vi "LTC change to stable temp.vi"(2 "Point Number":i32 min=-20 step=1, 3 "L:TC 21 Address":refnum<visa-resource-name>) -> (0 "Stop":bool, 1 "Stable temperature (K)":dbl[](array[numeric]) format="%.2f")   [LabVIEW 2025]
doc: "Changes the setpoint and waits for temperature to stablilize near the setpoint. Can set how stable and how close to the setpoint one wants the temperature to be. Allows changing of the PID parameters.\nMurali Chaparala, Scott Hannahs, NHMFL - FSU, November 1996\nAuthor: Scott Hannahs <sth@magnet.fsu.edu>\n\nThis software is licensed for use under the “MIT License\"\nCopyright (c) 2025 Scott Hannahs, sth@sth@magnet.sthnet.net\n\nPermission is hereby granted, free of charge, to any person obtaining a copy of this software and associated documentation files (the \"Software\"), to deal in the Software without restriction, including without limitation the rights to use, copy, modify, merge, publish, distribute, sublicense, and/or sell copies of the Software, and to permit persons to whom the Software is furnished to do so, subject to the following conditions: The above copyright notice and this permission notice shall be included in all copies or substantial portions of the Software.\n\nTHE SOFTWARE IS PROVIDED \"AS IS\", WITHOUT WARRANTY OF ANY KIND, EXPRESS OR IMPLIED, INCLUDING BUT NOT LIMITED TO THE WARRANTIES OF MERCHANTABILITY, FITNESS FOR A PARTICULAR PURPOSE AND NONINFRINGEMENT. IN NO EVENT SHALL THE AUTHORS OR COPYRIGHT HOLDERS BE LIABLE FOR ANY CLAIM, DAMAGES OR OTHER LIABILITY, WHETHER IN AN ACTION OF CONTRACT, TORT OR OTHERWISE, ARISING FROM, OUT OF OR IN CONNECTION WITH THE SOFTWARE OR THE USE OR OTHER DEALINGS IN THE SOFTWARE."
uses:
  <vilib>/Analysis/NI_AALBase.lvlib
panel:
  out "Power %":dbl format="%.2f"
  out "Current Temperature Profile":dbl[][](graph)
  in  "PID param":dbl[][](array[numeric])=[[1.0, 0.0, 0.0, 0.0], [1.0, 0.0, 0.0, 0.0]] format="%.3f"
  out "Temperature set points":dbl[](array[numeric]) format="%.2f"
  in  "File containing the temperature set points:":path
  in  "Use Sensor 2?":bool=TRUE
  in  "Difference between\nInner and outer temperature (K).":dbl=3.0 min=0.0 max=20.0 step=1.0 format="%.2f"
  in  "Number of data sets to read for each stable temperature?":i32=10 min=1 step=1
  in  "What is the % deviation\nof the STABLE, AVERAGE \nsample  temperature from\nthe set point that we \nconsider acceptable?":dbl min=0.0 format="%.3f"
  in  "What is the % variation of\nthe sample temperature \nabout the mean value that\nwe consider acceptable to\ndefine it as being stable?":dbl=0.01000000000000001 min=0.0 step=0.01 format="%.3f"
  in  "Number of points\nused to determine \nstable temperature.":i32=60 min=1 max=1000 step=1
  in  "DeltaT (ms)":u32=1000 max=3600000 step=10
  out "Time over which the stability criterion was satisfied (S).":dbl format="%.2f"
  out "Temperature Fluctuation \nabout the AVERAGE \nvalue (%).":dbl min=0.0 format="%.3f"
  out "% Deviation of the\nsample temperature\nfrom the set point.":dbl=0.001 min=0.001 max=310.0 format="%.3f"
  # "Sensor1 Panel"
  # "Sensor 2 Panel"
  # "Stability Panel"
  # "P"
  # "I"
  # "D"
  # "P0"
  # "Heater"
  # "Analog"
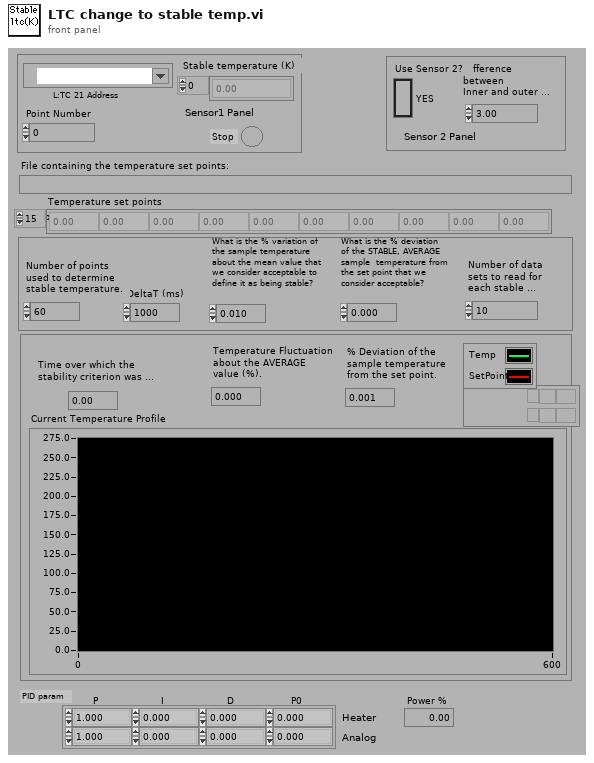
[diagram p1: front panel]
types:
  T1 = cluster{"X Minimum":dbl, "Number of points\nused to determine \nstable temperature.":i32, "X Maximum":dbl}
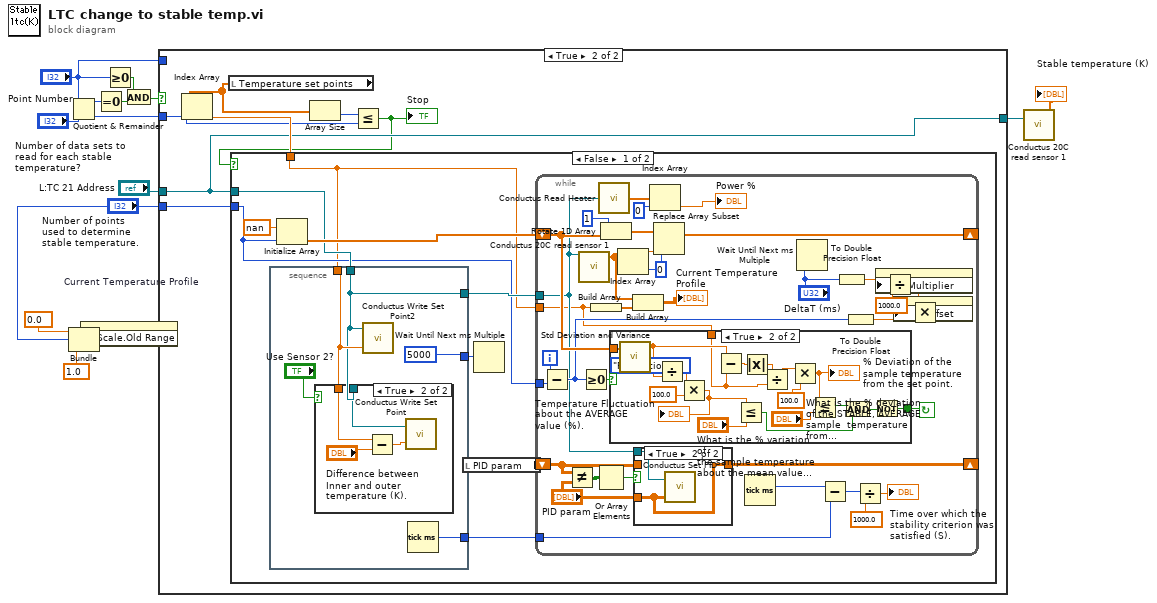
[diagram p0: block diagram]
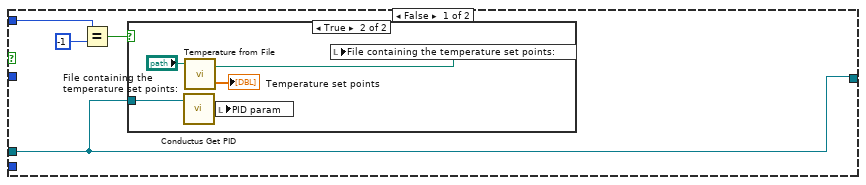
[diagram p2: hidden frame]
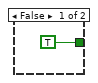
[diagram p5: hidden frame]
diagram:
  n1 = Quotient & Remainder(x="Point Number", y="Number of data sets to read for each stable temperature?") -> (x-y*floor(x/y)=w14:i32, floor(x/y)=w12:i32)
  n2 = Bundle("X Minimum"=0.0, "Number of points\nused to determine \nstable temperature."="Number of points\nused to determine \nstable temperature.", "X Maximum"=1.0) -> (w4:T1)  [unwired: 1 in]
  n3 = property on="Current Temperature Profile" class="WFChart (strict)"("X Scale.Old Range"=w4) -> ()  [unwired: 2 in, 2 out]
  n4 = Equal To 0?(x=w14) -> (x = 0?=w10:bool)
  n5 = Greater Or Equal To 0?(x="Point Number") -> (x >= 0?=w11:bool)
  n6 = And(x=w11, y=w10) -> (x .and. y?=w9:bool)
  n7 = case shown="True" w9 {
    tunnel: "L:TC 21 Address" -> [w15 w28]
    tunnel: "Number of points\nused to determine \nstable temperature." -> [_ w29]
    tunnel: w12 -> [_ w25]
    tunnel: [w15 w28] -> w7
    tunnel: "Point Number" -> [w17 _]
    frame False {
      n8 = Equal?(x=w17, y=-1) -> (x = y?=w16:bool)
      n9 = case shown="True" w16 {
        tunnel: w15 -> [_ w21]
        frame False {
        }
        frame True {
          n10 = call "Conductus Get PID.vi"("Instrument Address"=w21) -> ("PID Param"=w20:dbl[][])  [unwired: 1 in, 1 out]
          n11 = call "Temperature from File.vi"("File Name:"="File containing the temperature set points:") -> ("File Path"=w19:path, "Temperature set points"=→"Temperature set points":dbl[])
          n12 = local write "PID param"(w20) -> ()
          n13 = local write "File containing the temperature set points:"(w19) -> ()
        }
      }
    }
    frame True {
      n14 = local read "Temperature set points"() -> (w27:dbl[])
      n15 = Index Array(array=w27, index=w25) -> (element=w30:dbl)
      n16 = Array Size(array=w27) -> (size(s)=w26:i32)
      n17 = Less Or Equal?(x=w26, y=w25) -> (x <= y?=w24:bool)
      "Stop" <- w24
      n18 = case shown="False" w24 {
        tunnel: w30 -> [w31 _]
        tunnel: w28 -> [w35 _]
        tunnel: w29 -> [w34 _]
        frame False {
          n19 = stacked-sequence {
            tunnel: w35 -> [w99]
            tunnel: w31 -> [w102]
            tunnel: [u32 5000] -> w37
            tunnel: [w99] -> w36
            tunnel: [w98] -> w32
            frame #0 {
              n20 = case shown="True" "Use Sensor 2?" {
                tunnel: w102 -> [_ w105]
                tunnel: w99 -> [_ w103]
                frame False {
                }
                frame True {
                  n21 = Subtract(x=w105, y="Difference between\nInner and outer temperature (K).") -> (x-y=w104:dbl)
                  n22 = call "Conductus Write Set Point.vi"("Setpoint"=w104, "Instrument Address"=w103) -> ()  [unwired: 1 in]
                }
              }
              n23 = call "Conductus Write Set Point2.vi"("Setpoint"=w102, "GPIB Address"=w99) -> ()  [unwired: 1 in]
              n24 = Tick Count (ms)() -> (millisecond timer value=w98:u32)
            }
          }
          n25 = Initialize Array(nan, w34) -> (w39:dbl[])
          n26 = local read "PID param"() -> (w33:dbl[][])
          n27 = Wait Until Next ms Multiple(millisecond multiple=w37) -> ()  [unwired: 1 out]
          n28 = while {
            tunnel: w31 -> [w40]
            tunnel: w32 -> [w58]
            shift-left: w33 -> [w62]
            shift-right: [w61] -> _
            tunnel: w36 -> [w47]
            tunnel: w34 -> [w71]
            shift-left: w39 -> [w68]
            shift-right: [w45] -> _
            i -> [w70]
            stop <- w69 continue-if-true
            w74 = 0
            n29 = Subtract(x=w70, y=w71) -> (x-y=w54:i32)
            n30 = Not Equal?(x=w62, y="PID param") -> (x != y?=w64:bool[][])
            n31 = call "Conductus 20C read sensor 1.vi"("Instrument Address"=w47) -> ("Output"=w43:dbl[])  [unwired: 1 in, 1 out]
            n32 = Greater Or Equal To 0?(x=w54) -> (x >= 0?=w55:bool)
            n33 = Build Array(w40) -> (w41:dbl[])
            n34 = Or Array Elements(Boolean array=w64) -> (logical OR=w63:bool)
            n35 = call "Conductus Read Heater.vi"("Instrument Address"=w47) -> ("Heater Power %"=w49:dbl[])
            n36 = Rotate 1D Array(1:w68, 2:1) -> (0:w73:dbl[])
            n37 = case shown="True" w55 {
              tunnel: [TRUE w80] -> w69
              tunnel: w68 -> [_ w82]
              tunnel: w40 -> [_ w81]
              frame False {
              }
              frame True {
                n38 = call <vilib>:"Std Deviation and Variance.vi"("X"=w82, "Weighting (Sample)"=enum16{"Sample", "Population"}."Population") -> ("mean"=w95:dbl, "standard deviation"=w94:dbl)  [unwired: 1 out]
                n39 = Divide(x=w94, y=w95) -> (x/y=w88:dbl)
                n40 = Multiply(x=w88, y=100.0) -> (x*y=w96:dbl)
                "Temperature Fluctuation \nabout the AVERAGE \nvalue (%)." <- w96
                n41 = Subtract(x=w95, y=w81) -> (x-y=w83:dbl)
                n42 = Less Or Equal?(x=w96, y="What is the % variation of\nthe sample temperature \nabout the mean value that\nwe consider acceptable to\ndefine it as being stable?") -> (x <= y?=w91:bool)
                n43 = Absolute Value(x=w83) -> (abs(x)=w84:dbl)
                n44 = Divide(x=w84, y=w81) -> (x/y=w85:dbl)
                n45 = Multiply(x=w85, y=100.0) -> (x*y=w93:dbl)
                "% Deviation of the\nsample temperature\nfrom the set point." <- w93
                n46 = Less Or Equal?(x=w93, y="What is the % deviation\nof the STABLE, AVERAGE \nsample  temperature from\nthe set point that we \nconsider acceptable?") -> (x <= y?=w97:bool)
                n47 = And(x=w97, y=w91) -> (x .and. y?=w92:bool)
                n48 = Not(x=w92) -> (.not. x?=w80:bool)
              }
            }
            n49 = Index Array(array=w43, index=w74) -> (element=w44:dbl)
            n50 = Build Array(w43, w41) -> (→"Current Temperature Profile":dbl[][])
            n51 = case shown="True" w63 {
              tunnel: "PID param" -> [_ w77]
              tunnel: [w75 w77] -> w61
              tunnel: w62 -> [w75 _]
              tunnel: w47 -> [_ w76]
              frame False {
              }
              frame True {
                n52 = call "Conductus Set PID.vi"("PID param"=w77, "Instrument Address"=w76) -> ()  [unwired: 1 in, 1 out]
              }
            }
            n53 = Index Array(array=w49, index=0 ("Index")) -> (element=→"Power %":dbl)
            n54 = Replace Array Subset(array=w73, new element=w44, index=w74) -> (w45:dbl[])
            n55 = Tick Count (ms)() -> (millisecond timer value=w56:u32)
            n56 = Wait Until Next ms Multiple(millisecond multiple="DeltaT (ms)") -> ()  [unwired: 1 out]
            n57 = Subtract(x=w56, y=w58) -> (x-y=w57:u32)
            n58 = To Double Precision Float(number="DeltaT (ms)") -> (double precision float=w50:dbl)
            n59 = To Double Precision Float(number=w54) -> (double precision float=w51:dbl)
            n60 = Divide(x=w57, y=1000.0) -> (x/y=→"Time over which the stability criterion was satisfied (S).":dbl)
            n61 = Divide(x=w50, y=1000.0) -> (x/y=w53:dbl)
            n62 = property on="Current Temperature Profile" class="WFChart (strict)"("X Scale.Offset and Multiplier:Multiplier"=w53) -> ()  [unwired: 2 in, 2 out]
            n63 = Multiply(x=w53, y=w51) -> (x*y=w52:dbl)
            n64 = property on="Current Temperature Profile" class="WFChart (strict)"("X Scale.Offset and Multiplier:Offset"=w52) -> ()  [unwired: 2 in, 2 out]
          }
        }
        frame True {
        }
      }
    }
  }
  n65 = call "Conductus 20C read sensor 1.vi"("Instrument Address"=w7) -> ("Output"=→"Stable temperature (K)":dbl[])  [unwired: 1 in, 1 out]
